vi "Conductus Get Data.vi"(2 "Point #":i32, 3 "Command String":string, 4 "GPIB Address":refnum<visa-resource-name>) -> (0 "Stop":bool, 1 "Measurement":dbl[](array[numeric]) format="%.2e")   [LabVIEW 2025]
doc: "This VI reads a single reading from a Keithley 2001 multimeter. The stop boolean is always false. If no reading is obtained a single zero is returned.\nScott Hannahs, NHMFL-FSU, Nov 1993 \nAuthor: Scott Hannahs <sth@magnet.fsu.edu>\n\nThis software is licensed for use under the “MIT License\"\nCopyright (c) 2025 Scott Hannahs, sth@sth@magnet.sthnet.net\n\nPermission is hereby granted, free of charge, to any person obtaining a copy of this software and associated documentation files (the \"Software\"), to deal in the Software without restriction, including without limitation the rights to use, copy, modify, merge, publish, distribute, sublicense, and/or sell copies of the Software, and to permit persons to whom the Software is furnished to do so, subject to the following conditions: The above copyright notice and this permission notice shall be included in all copies or substantial portions of the Software.\n\nTHE SOFTWARE IS PROVIDED \"AS IS\", WITHOUT WARRANTY OF ANY KIND, EXPRESS OR IMPLIED, INCLUDING BUT NOT LIMITED TO THE WARRANTIES OF MERCHANTABILITY, FITNESS FOR A PARTICULAR PURPOSE AND NONINFRINGEMENT. IN NO EVENT SHALL THE AUTHORS OR COPYRIGHT HOLDERS BE LIABLE FOR ANY CLAIM, DAMAGES OR OTHER LIABILITY, WHETHER IN AN ACTION OF CONTRACT, TORT OR OTHERWISE, ARISING FROM, OUT OF OR IN CONNECTION WITH THE SOFTWARE OR THE USE OR OTHER DEALINGS IN THE SOFTWARE."
panel:
  in  "Eng Units?":bool
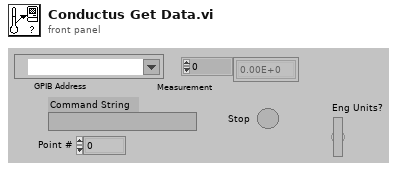
[diagram p1: front panel]
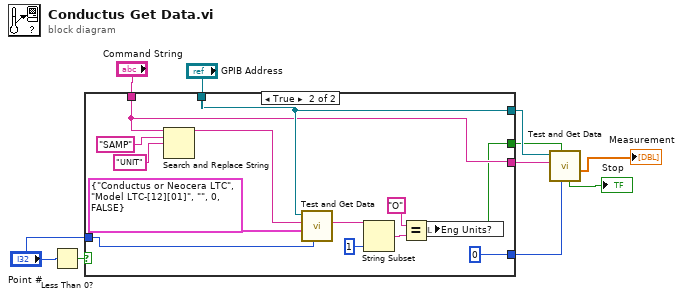
[diagram p0: block diagram]
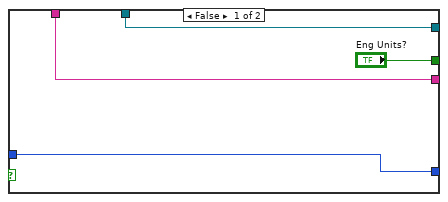
[diagram p2: hidden frame]
diagram:
  n1 = Less Than 0?(x="Point #") -> (x < 0?=w8:bool)
  n2 = case shown="True" w8 {
    tunnel: "Point #" -> [w12 w27]
    tunnel: "Command String" -> [w13 w17]
    tunnel: "GPIB Address" -> [w14 w18]
    tunnel: [w14 w18] -> w6
    tunnel: [w13 w17] -> w4
    tunnel: [w12 0] -> w3
    tunnel: ["Eng Units?" w15] -> w1
    frame False {
    }
    frame True {
      n3 = Search and Replace String(input string=w17, search string="SAMP", replace string="UNIT" ("replace string (\"\")")) -> (result string=w23:string)  [unwired: 5 in, 3 out]
      n4 = call "Test and Get Data.vi"("Point #"=w27, "Instrument Info"=cluster{string, string, string, u32, bool} {"Conductus or Neocera LTC", "Model LTC-[12][01]", "", 0, FALSE}, "Command String"=w23, "VISA Sesson"=w18) -> ("String Response"=w22:string)  [unwired: 2 in, 4 out]
      n5 = String Subset(string=w22, length (rest)=1 ("length (rest)")) -> (substring=w20:string)  [unwired: 1 in]
      n6 = Equal?(x="O", y=w20) -> (x = y?=w15:bool)
      n7 = local write "Eng Units?"(w15) -> ()
    }
  }
  n8 = call "Test and Get Data.vi"("Point #"=w3, "Eng Units?"=w1, "Command String"=w4, "VISA Sesson"=w6) -> ("Measurement"=→"Measurement":dbl[], "Stop"=→"Stop":bool)  [unwired: 2 in, 3 out]
